vi "case duplicator.vi"   [LabVIEW 2013]
uses:
  <vilib>/Utility/traverseref.llb/TRef TravTarget.ctl
  tag bus/trunk/tag/Data Type.ctl
  tag bus/trunk/dictionary/create group specification.vi
  <vilib>/Utility/traverseref.llb/VI Scripting - Traverse.lvlib
  tag bus/trunk/tag/tag descriptor.lvclass
  <vilib>/Utility/VariantDataType/VariantType.lvlib
  tag bus/trunk/dictionary/data dictionary.lvclass
types:
  T1 = typedef "TRef TravTarget.ctl" = enum16{"FP", "BD", "Other"}
  T2 = typedef "tag bus.lvlib/tag descriptor.lvclass/Data Type.ctl" = enum16{"Double", "Single", "I64", "I32", "I16", "I8", "U64", "U32", "U16", "U8", "Boolean", "String", "Array of Double", "Array of Single", "Array of I64", "Array of I32", "Array of I16", "Array of I8", "Array of U64", "Array of U32", "Array of U16", "Array of U8", "Array of Boolean", "Array of String"}
  T3 = typedef "VariantType.lvlib/Type.ctl" = enum8{"Invalid Type", "Void", "I8", "I16", "I32", "I64", "U8", "U16", "U32", "U64", "Single Float", "Double Float", "Extended Float", "Single Complex", "Double Complex", "Extended Complex", "Enum U8", "Enum U16", "Enum U32", "Enum U64", "Single Float With Unit", "Double Float With Unit", "Extended Float With Unit", "Single Complex with Unit", "Double Complex with Unit", "Extended Complex with Unit", "Boolean", "String", "Path", "Picture", "Tag", "Array", "Cluster", "Variant", "LV Variant", "Waveform", "Timestamp", "Digital Waveform", "Digital Data", "ExpressData", "Refnum", "External Data", "VI", "Poly VI", "LabVIEW Class Instance", "Fixed Point"}
  T4 = typedef "VariantType.lvlib/TypedefInfo.ctl" = cluster{"Name":string, "Timestamp":u32}
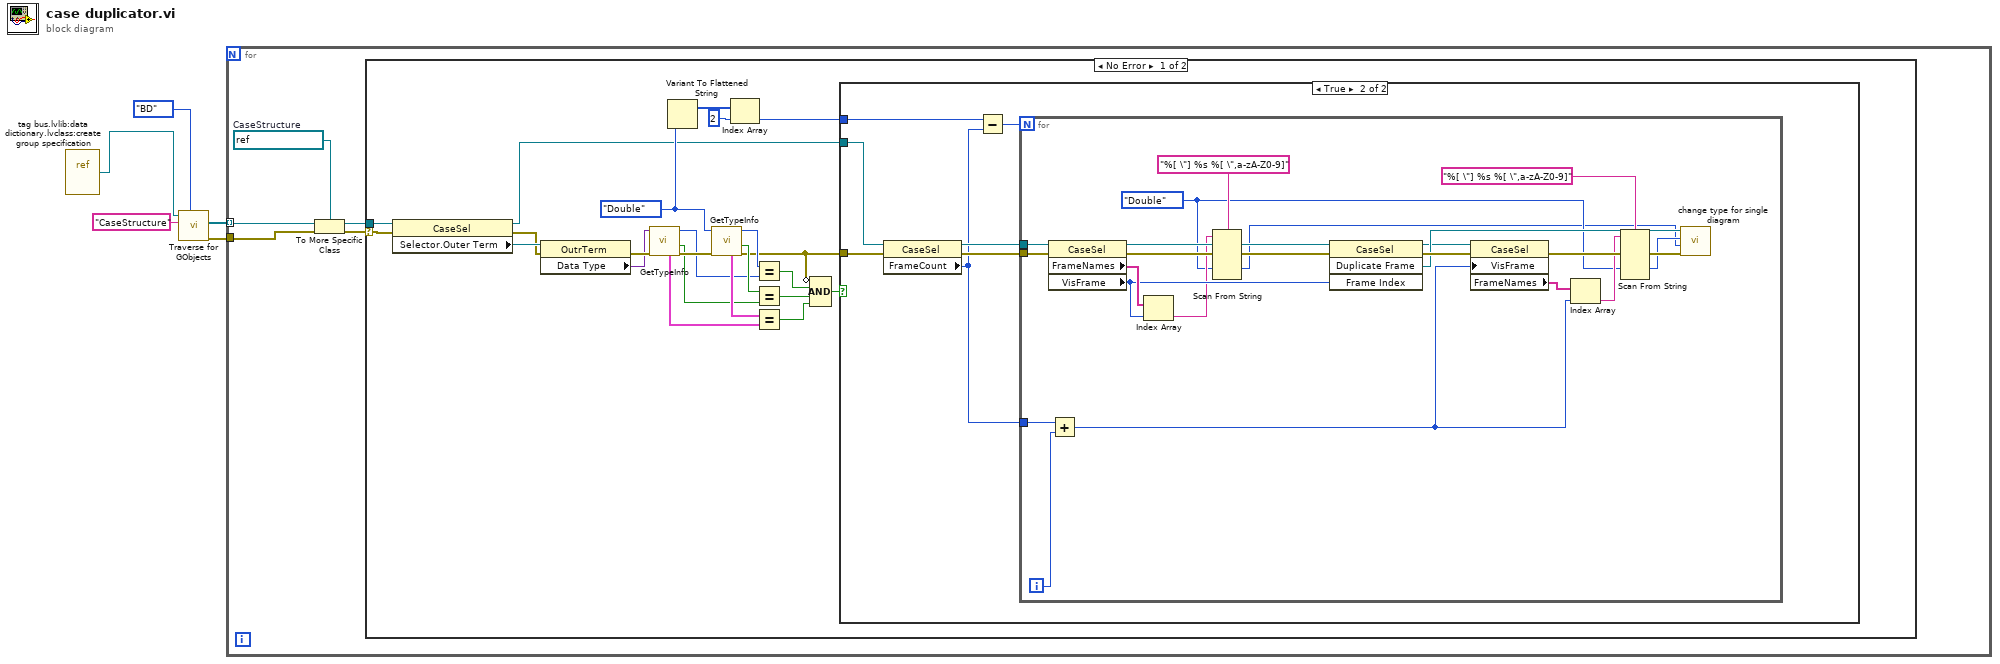
[diagram p0: block diagram]
diagram:
  n1 = vi-ref "tag bus.lvlib:data dictionary.lvclass:create group specification.vi"() -> (w1:refnum<vi>)
  n2 = call <vilib>:"Traverse for GObjects.vi"("Traverse Target"=TRef_TravTarget."BD", "Class Name"="CaseStructure", "VI Refnum"=w1) -> ("error out"=w2:errorcluster, "References"=w3:refnum<vi>[])  [unwired: 5 in, 2 out]
  n3 = for {
    tunnel: w3 -> [w10] mode=indexing
    tunnel: w2 -> [w8]
    w9 = refnum<vi> refnum  # CaseStructure
    n4 = To More Specific Class(target class=w9, reference=w10, error in=w8) -> (specific class reference=w6:refnum<vi>, error out=w7:errorcluster)
    n5 = case shown="No Error" w7 {
      selector: w7 -> [w32 _]
      tunnel: w6 -> [w33 _]
      frame No Error {
        w14 = Data_Type."Double" ("Data Type")
        n6 = property class="CaseSel"(reference=w33, error in=w32) -> (reference out=w11:refnum<vi>, error out=w30:errorcluster, "Selector.Outer Term"=w31:refnum<vi>)
        n7 = property class="OutrTerm"(reference=w31, error in=w30) -> (error out=w29:errorcluster, "Data Type"=w28:variant)  [unwired: 1 out]
        n8 = call <vilib>:"GetTypeInfo.vi"("error in (no error)"=w29, "Variant"=w28) -> ("error out"=w27:errorcluster, "HasTypedef"=w19:bool, "Type Enum"=w18:T3, "TypedefInfo"=w25:T4)  [unwired: 5 in, 1 out]
        n9 = Variant To Flattened String(Variant=w14) -> (1:w15:i16[])  [unwired: 1 out]
        n10 = call <vilib>:"GetTypeInfo.vi"("error in (no error)"=w27, "Variant"=w14) -> ("error out"=w12:errorcluster, "HasTypedef"=w20:bool, "Type Enum"=w21:T3, "TypedefInfo"=w26:T4)  [unwired: 5 in, 1 out]
        n11 = Index Array(array=w15, index=2) -> (element=w13:i16)
        n12 = Equal?(x=w21, y=w18) -> (x = y?=w22:bool)
        n13 = Equal?(x=w20, y=w19) -> (x = y?=w24:bool)
        n14 = Equal?(x=w26, y=w25) -> (x = y?=w23:bool)
        n15 = Compound Arithmetic op=AND(invert w12, w22, w24, w23) -> (w17:bool)
        n16 = case shown="True" w17 {
          tunnel: w13 -> [_ w38]
          tunnel: w12 -> [_ w39]
          tunnel: w11 -> [_ w40]
          frame False {
          }
          frame True {
            n17 = property class="CaseSel"(reference=w40, error in=w39) -> (reference out=w36:refnum<vi>, error out=w35:errorcluster, "FrameCount"=w34:i32)
            n18 = Subtract(x=w38, y=w34) -> (x-y=w37:i32)
            n19 = for {
              N: w37 -> [_]
              tunnel: w36 -> [w63]
              tunnel: w35 -> [w62]
              tunnel: w34 -> [w49]
              i -> [w48]
              w43 = Data_Type."Double" ("Data Type")
              n20 = property class="CaseSel"(reference=w63, error in=w62) -> (reference out=w59:refnum<vi>, error out=w60:errorcluster, "FrameNames"=w61:string[], "VisFrame"=w58:u32)
              n21 = Add(x=w49, y=w48) -> (x+y=w46:i32)
              n22 = Index Array(array=w61, index=w58) -> (element=w53:string)
              n23 = Scan From String(format string="%[ \"] %s %[ \",a-zA-Z0-9]", input string=w53, error in=w60, default 2=w43) -> (error out=w54:errorcluster, output 2=w41:T2)  [unwired: 5 in, 2 out]
              n24 = invoke class="CaseSel" method="Duplicate Frame"(reference=w59, error in=w54, "Frame Index"=w58) -> (reference out=w50:refnum<vi>, error out=w57:errorcluster, "Duplicate Frame"=w55:refnum<vi>)  [unwired: 1 in, 1 out]
              n25 = property class="CaseSel"(reference=w50, error in=w57, "VisFrame"=w46) -> (error out=w56:errorcluster, "FrameNames"=w47:string[])  [unwired: 1 out]
              n26 = Index Array(array=w47, index=w46) -> (element=w51:string)
              n27 = Scan From String(format string="%[ \"] %s %[ \",a-zA-Z0-9]", input string=w51, error in=w56, default 2=w43) -> (error out=w52:errorcluster, output 2=w42:T2)  [unwired: 5 in, 2 out]
              n28 = call "change type for single diagram.vi"("error in (no error)"=w52, "old type"=w41, "new type"=w42, "Diagram in"=w55) -> ()  [unwired: 8 in]
            }
          }
        }
      }
      frame Error {
      }
    }
  }
